vi "globalVariables.vi"() -> ()   [LabVIEW 2023]
panel:
  out "System user":string
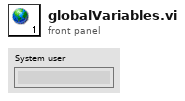
[diagram p1: front panel]
diagram:
